vi "QTrkTest.vi"() -> ()   [LabVIEW 2011]
uses:
  QTrk.llb/QTrkSettings.ctl
  QTrk.llb/QTrkDLL.vi
panel:
  in  "QTrk Settings":T1={"Image width"=150, "Image height"=150, "Number of threads (CPU based)"=-1, "XCOR Profile Length"=128, "XCOR Profile Width"=32, "XCOR Iterations"=2, "ZLUT MinRadius"=5.0, "ZLUT MaxRadius"=50.0, "ZLUT AngularSteps"=64, "QI Iterations"=0, "QI RadialSteps"=64, "QI AngularSteps"=64, "QI MinRadius"=2.0, "QI MaxRadius"=50.0}
  in  "QTrk DLL":path
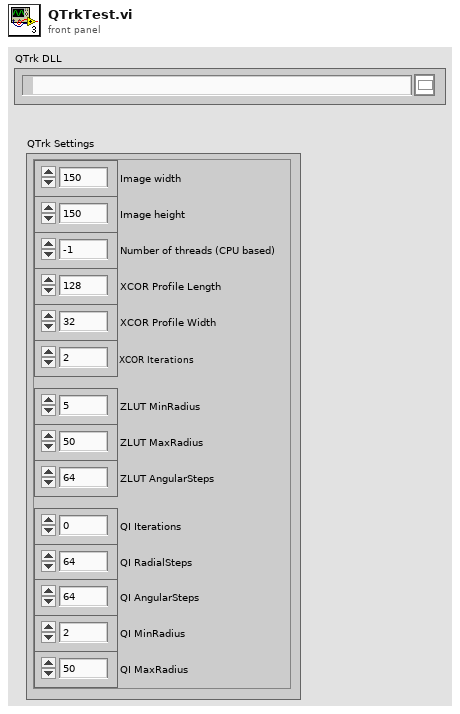
[diagram p1: front panel]
types:
  T1 = typedef "QTrkSettings.ctl" = cluster{"Image width":i32, "Image height":i32, "Number of threads (CPU based)":i32, "XCOR Profile Length":i32, "XCOR Profile Width":i32, "XCOR Iterations":i32, "ZLUT MinRadius":sgl, "ZLUT MaxRadius":sgl, "ZLUT AngularSteps":i32, "QI Iterations":i32, "QI RadialSteps":i32, "QI AngularSteps":i32, "QI MinRadius":sgl, "QI MaxRadius":sgl}
  T2 = typedef "QTrkInstance.ctl" = cluster{"QTrk Pointer":u64, "QTrk Settings":T1}
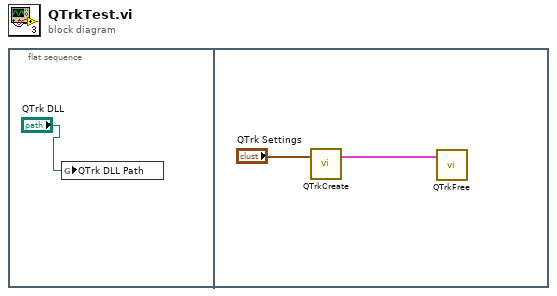
[diagram p0: block diagram]
diagram:
  n1 = flat-sequence {
    frame #0 {
      n2 = global write "QTrkDLL.vi" "QTrk DLL Path"("QTrk DLL") -> ()
    }
    frame #1 {
      n3 = call "QTrkCreate.vi"("QTrk Settings"="QTrk Settings") -> ("QTrk Instance"=w2:T2)  [unwired: 2 in]
      n4 = call "QTrkFree.vi"("QTrk Instance"=w2) -> ()  [unwired: 2 in]
    }
  }
